vi "Main.vi"(11 "Module Admin":refnum<class "Delacor_lib_QMH_Module Admin.lvclass">) -> ()   [LabVIEW 2023, in "Graph_data_collector.lvlib"]
doc: "This template is based off of the Queued Message Handler design pattern and the Queued Message Handler project template that ships with LabVIEW.\n\nThe main difference is that the queue is private to this module and communication between modules is performed via Broadcast and Request events.\n\nRequest events are wrapped in public API methods and are handled in the Event Handling Loop (EHL) of this VI. Any module can register for Broadcast events sent by this module. The EHL generates messages based on user interface actions.\n\nThe Message Handling Loop (MHL) processes messages generated by the EHL, or by other messages. The messages are string values, so new messages can be added easily to the Message Cases case structure in the MHL. Each message cluster can also provide an optional value for Message Data, which is a variant that can be converted to whatever message-specific data is required.\n_____\nBased on DQMH Project Template 6.1.0.94."
uses:
  Graph_data_collector.lvlib
  <vilib>/Delacor/Delacor QMH/Libraries/Module Admin_class/Delacor_lib_QMH_Module Admin.lvclass
  Data Control.ctl
  Module Data--cluster.ctl
  <vilib>/Delacor/Delacor QMH/Libraries/Message Queue_class/Delacor_lib_QMH_Message Queue.lvclass/Delacor_lib_QMH_Message Queue.ctl
  Stop Argument--cluster.ctl
  <vilib>/Delacor/Delacor QMH/Libraries/Module Admin_class/Delacor_lib_QMH_Module Admin.lvclass/Delacor_lib_QMH_Module Admin.ctl
  New_Data Argument--cluster.ctl
  <vilib>/Utility/miscctls.llb/LVPointTypeDef.ctl
  Graph_UI/Module Data--cluster.ctl
  <vilib>/Delacor/Delacor QMH/Libraries/Message Queue_class/Delacor_lib_QMH_Enqueue Message (Single).vi
  <vilib>/Delacor/Delacor QMH/Libraries/Module Admin_class/Delacor_lib_QMH_Get External Launch.vi
  <vilib>/Utility/error.llb/Error Cluster From Error Code.vi
  <vilib>/ErrorRing/Error Ring.xnode
  <vilib>/Delacor/Delacor QMH/Libraries/Message Queue_class/Delacor_lib_QMH_Message Queue.lvclass
  Graph_UI/Graph_UI.lvlib
  Registration/Registration.lvlib
panel:
  in  "Data Type":T1 {"ЦАП, градС" format="%.3g"; "Тнагр, градС" format="%.3g"; "Q, мл" format="%.3g"; "Рдм, МПа" format="%.3g"; "Vпл, см3" format="Р2 %#.2f МПа"; "Рэфф, МПа" format="%.3g"; "dL, мм" format="%.4f"; "R, Ом" format="%.4f"; "Ргор, МПа" format="%.2f град.С"; "Рпл2, МПа" format="Р2 %#.2f МПа"; "Рпл1, МПа" format="Р2 %#.2f МПа"}
  in  "Clear_data":bool
  in  "Timeout":dbl=1.0 caption="Период" min=0.01 max=999.0 step=1.0 format="Период регистрации: %#.1f сек"
  in  "Select_OY":i32[](listbox)=[1] caption="Ось Y"
  in  "Select_OX":i32(listbox) caption="Ось Х"
  in  "Create_graph":bool
  out "error out":errorcluster
  out "Status":string
  in  "Simulate MHL Error":bool
  in  "Simulate EHL Error":bool
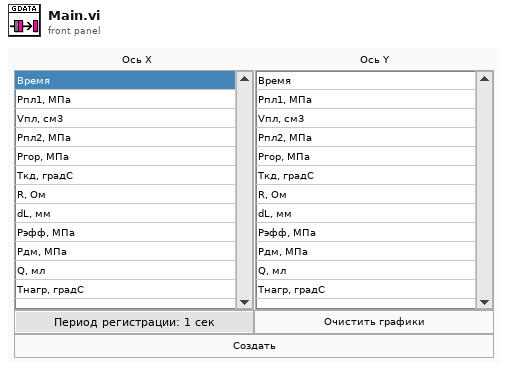
[diagram p1: front panel]
types:
  T1 = typedef "Graph_data_collector.lvlib/Data Control.ctl" = cluster{"Время":dbl, "Рпл1, МПа":dbl, "Vпл, см3":dbl, "Рпл2, МПа":dbl, "Ргор, МПа":dbl, "Ткд, градС":dbl, "R, Ом":dbl, "dL, мм":dbl, "Рэфф, МПа":dbl, "Рдм, МПа":dbl, "Q, мл":dbl, "Тнагр, градС":dbl, "ЦАП, градС":dbl}
  T2 = typedef "Graph_data_collector.lvlib/Request Events--cluster.ctl" = cluster{"Stop Module":refnum<user-event>, "Show Panel":refnum<user-event>, "Hide Panel":refnum<user-event>, "Get Module Execution Status":refnum<user-event>, "Show Diagram":refnum<user-event>, "New_Data":refnum<user-event>}
  T3 = typedef "Graph_data_collector.lvlib/Graph_UI.lvlib/Broadcast Events--cluster.ctl" = cluster{"Module Did Init":refnum<user-event>, "Status Updated":refnum<user-event>, "Error Reported":refnum<user-event>, "Module Did Stop":refnum<user-event>, "Update Module Execution Status":refnum<user-event>}
  T4 = typedef "Graph_data_collector.lvlib/Module Data--cluster.ctl" = cluster{"Status":string, "Array Lable":string[], "appended array":T1[], "Order Size":u32, "Graf_data_ref":refnum<vi>, "Actual_Data":T1}
  T5 = enum32{"invalid lock state", "Not Locked", "Locked (No Password)", "Password-protected"}
  T6 = typedef "Graph_data_collector.lvlib/Stop Argument--cluster.ctl" = cluster{"Origin":string, "Exit via Stop Module Req?":bool, "Wait for Module to stop?":bool}
  T7 = typedef "Graph_data_collector.lvlib/New_Data Argument--cluster.ctl" = cluster{"Graph_Data":T1}
  T8 = typedef "LVPointTypeDef.ctl" = cluster{"Horizontal":i16, "Vertical":i16}
  T9 = enum32{"Invalid", "Standard", "Closed", "Hidden", "Minimized", "Maximized"}
  T10 = typedef "Graph_data_collector.lvlib/Graph_UI.lvlib/Module Data--cluster.ctl" = cluster{"Status":string, "XY Graph our ref":refnum<vi>, "Array Lable":string[], "Ось Y":i32[], "Ось Х":i32, "Graph size":i32, "appended array":T1[], "XY Graph ref":refnum<vi>}
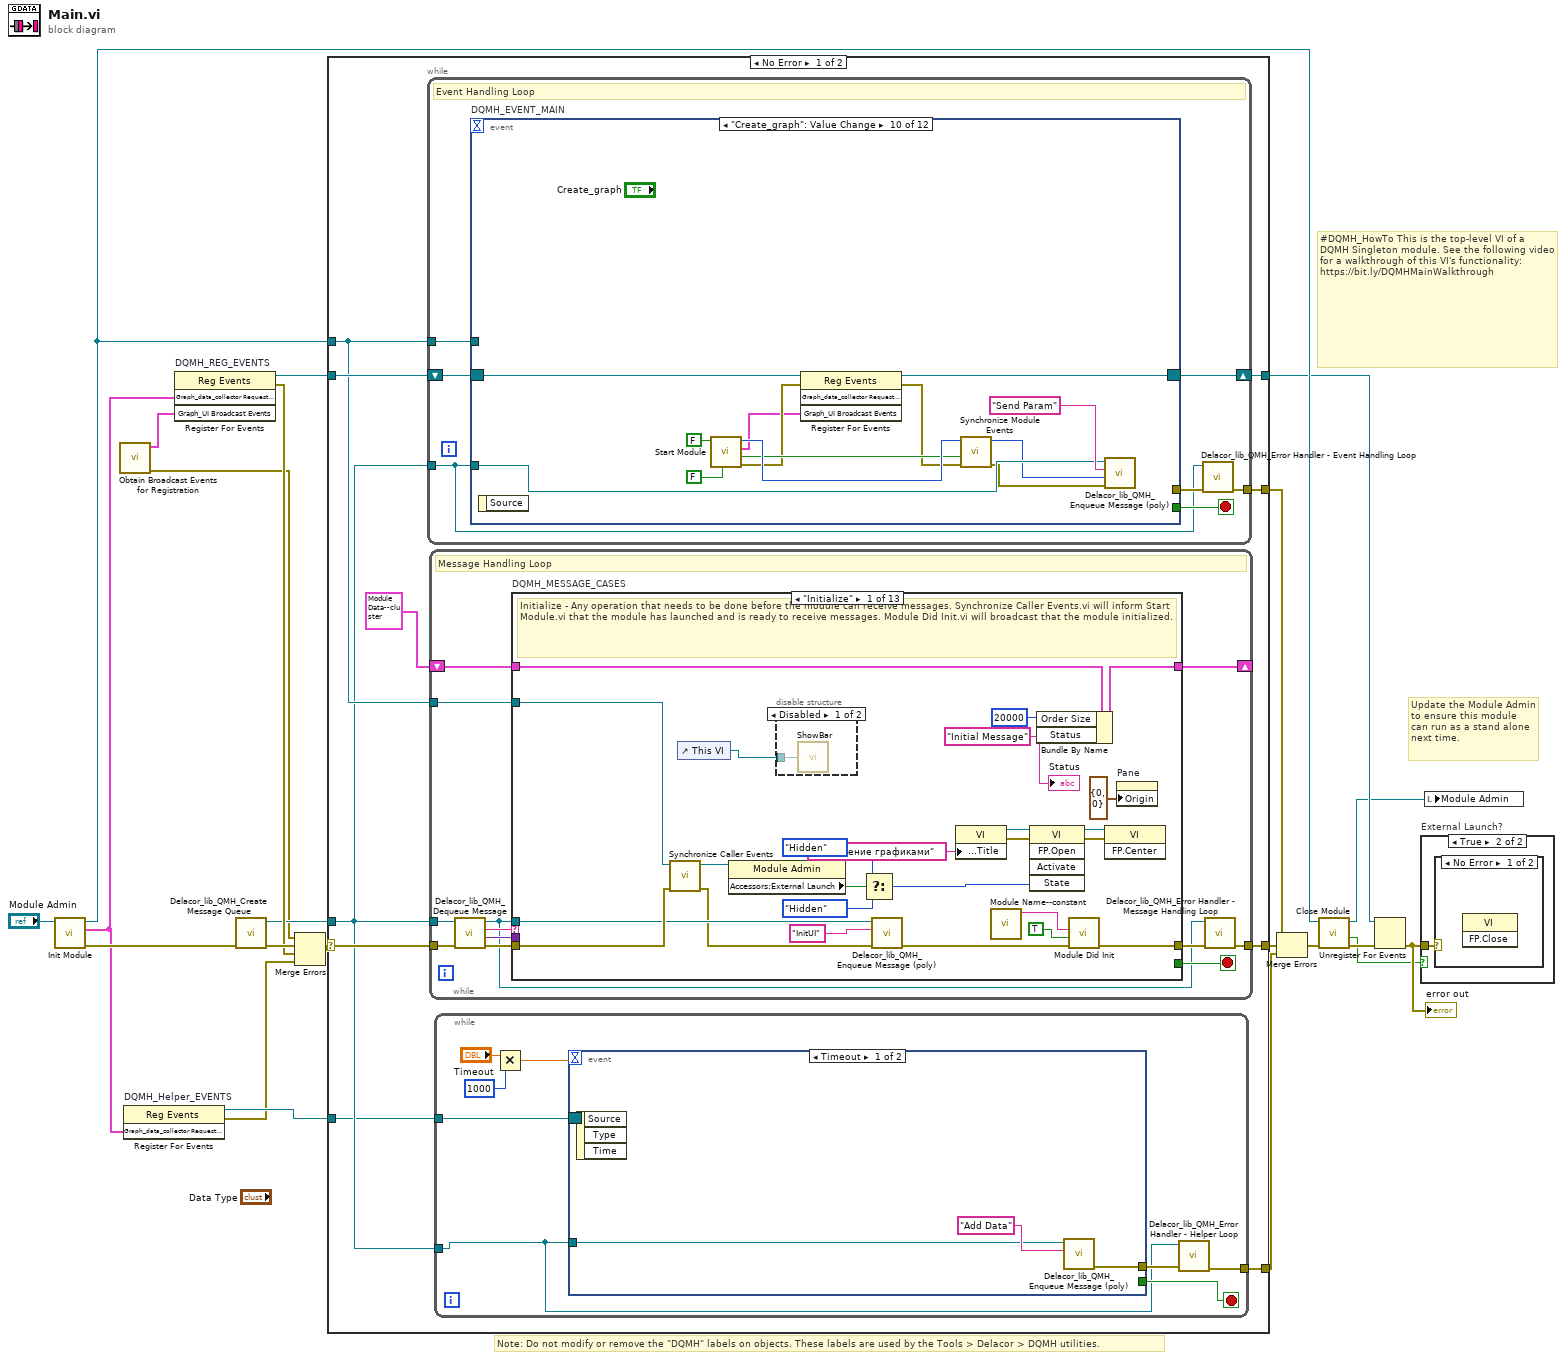
[diagram p0: block diagram]
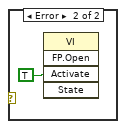
[diagram p3: hidden frame]
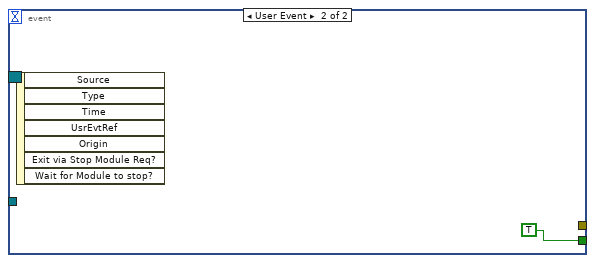
[diagram p4: hidden frame]
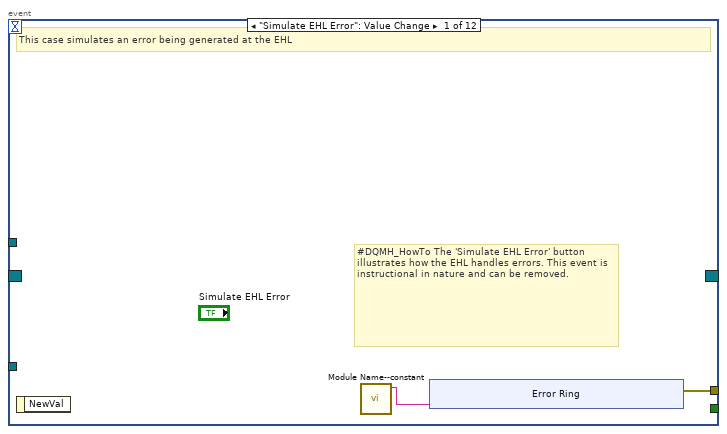
[diagram p5: hidden frame]
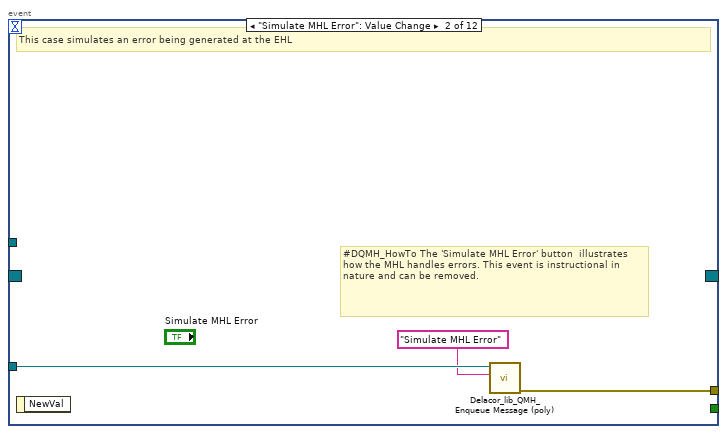
[diagram p6: hidden frame]
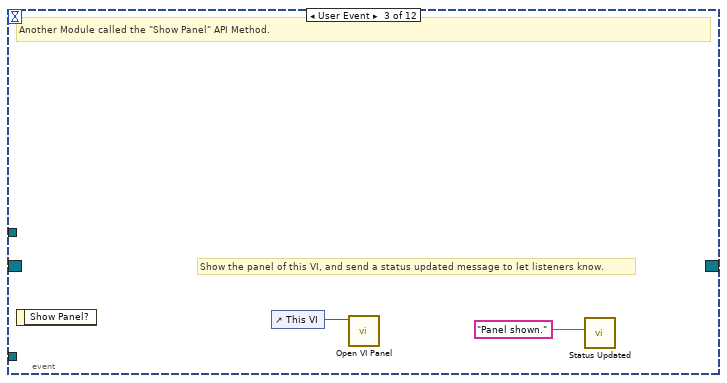
[diagram p7: hidden frame]
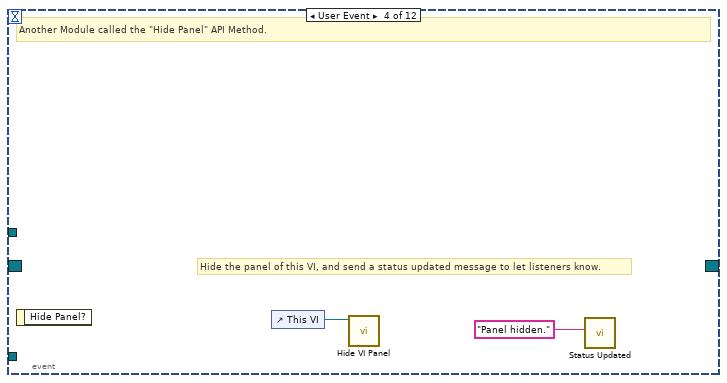
[diagram p8: hidden frame]
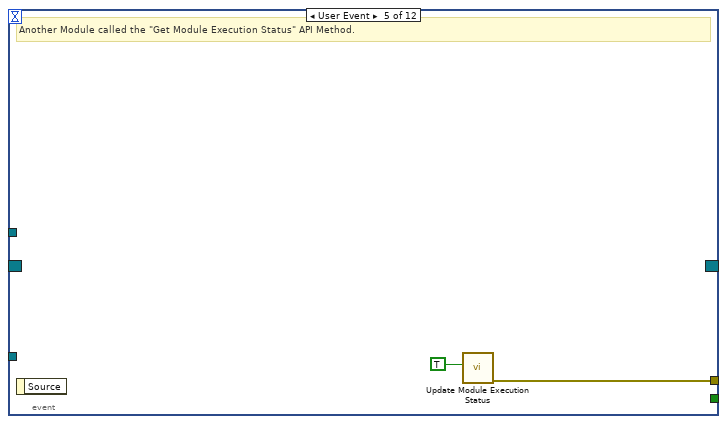
[diagram p9: hidden frame]
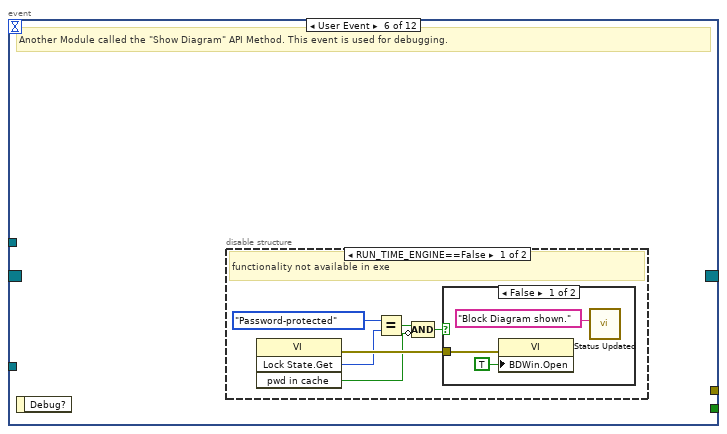
[diagram p10: hidden frame]
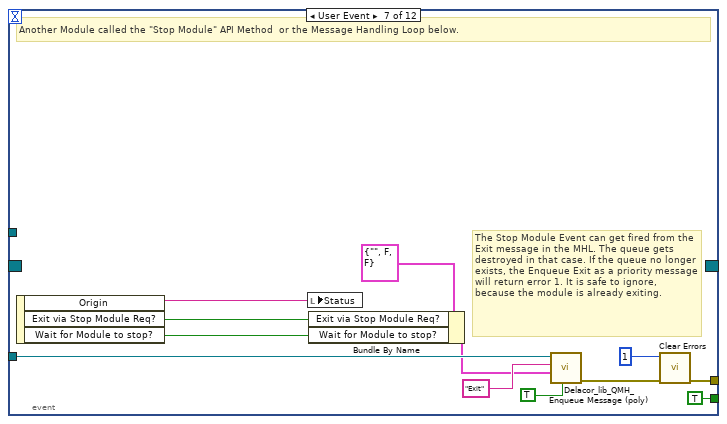
[diagram p13: hidden frame]
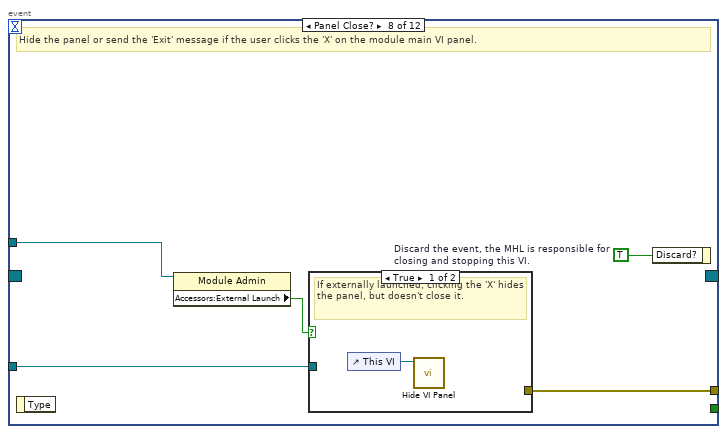
[diagram p14: hidden frame]
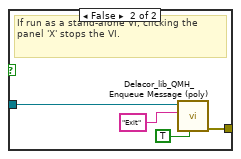
[diagram p15: hidden frame]
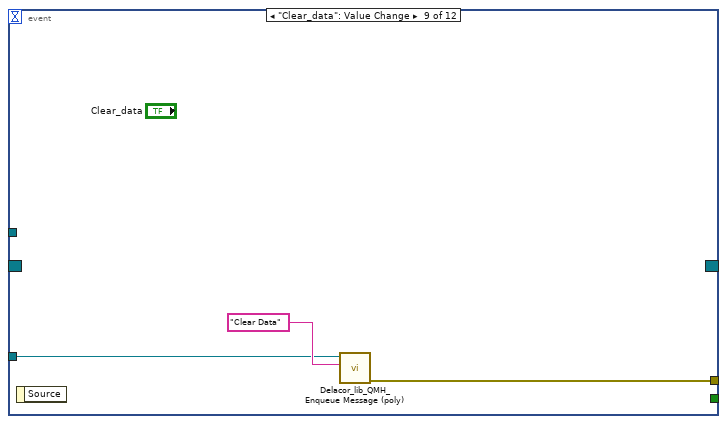
[diagram p16: hidden frame]
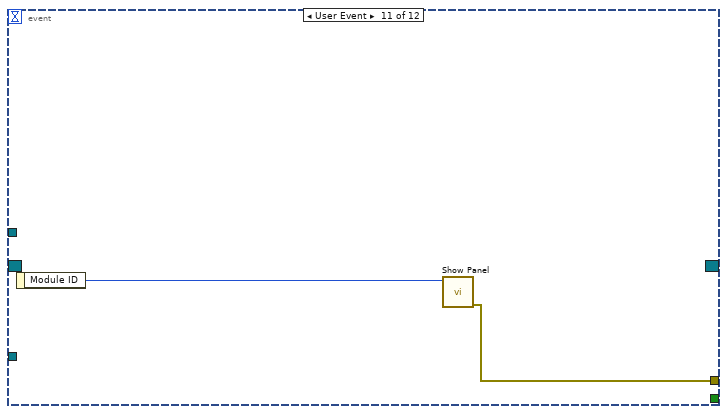
[diagram p17: hidden frame]
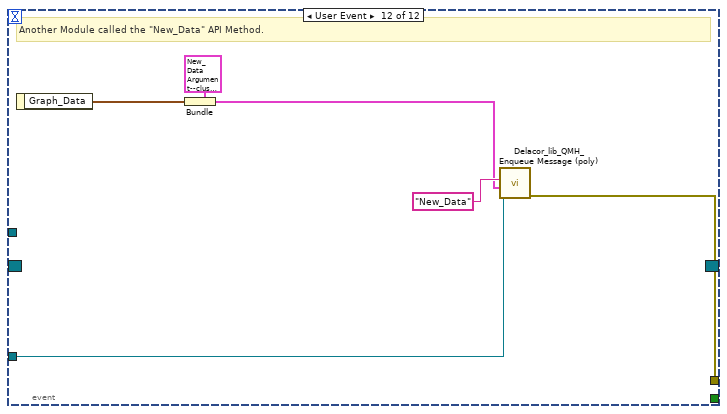
[diagram p18: hidden frame]
diagram:
  # "#DQMH_HowTo This is the top-level VI of a DQMH Singleton module. See the following video for a walkthrough of this VI's functionality: https://bit.ly/DQMHMainWalkthrough"
  # "Note: Do not modify or remove the \"DQMH\" labels on objects. These labels are used by the Tools > Delacor > DQMH utilities."
  # "Update the Module Admin to ensure this module can run as a stand alone next time."
  n1 = call "Init Module.vi"("Singleton Module Admin in"="Module Admin") -> ("error out"=w21:errorcluster, "Graph_data_collector Request Events"=w2:T2, "Singleton Module Admin out"=w13:refnum<class "Delacor_lib_QMH_Module Admin.lvclass">)  [unwired: 8 in]
  n2 = call "Obtain Broadcast Events for Registration.vi"() -> ("error out"=w5:errorcluster, "Graph_UI Broadcast Events"=w6:T3)  [unwired: 9 in, 1 out]
  n3 = register-events "DQMH_Helper_EVENTS"(w2) -> (reference out=w3:refnum<event-registration>, error out=w1:errorcluster)  [unwired: 2 in]
  n4 = register-events "DQMH_REG_EVENTS"(w2, w6) -> (reference out=w11:refnum<event-registration>, error out=w14:errorcluster)  [unwired: 2 in]
  n5 = call <vilib>:"Delacor_lib_QMH_Create Message Queue.vi"("error in"=w21) -> ("error out"=w16:errorcluster, "Message Queue"=w10:refnum<class "Delacor_lib_QMH_Message Queue.lvclass">)  [unwired: 9 in]
  n6 = Merge Errors(w5, w16, w14, w1) -> (w15:errorcluster)
  n7 = case shown="No Error" w15 {
    selector: w15 -> [w30 w288]
    tunnel: [w32 w287] -> w22
    tunnel: [w29 w293] -> w12
    tunnel: w11 -> [w28 w293]
    tunnel: w10 -> [w24 w286]
    tunnel: [w31 _] -> w19
    tunnel: w13 -> [w27 w289]
    tunnel: [w25 _] -> w4
    tunnel: w3 -> [w23 _]
    frame No Error {
      n8 = while {
        tunnel: w24 -> [w45]
        shift-right: [w48] -> w29
        shift-left: w28 -> [w49]
        tunnel: [w50] -> w31
        tunnel: w27 -> [w46]
        stop <- w47 stop-if-true
        # "Event Handling Loop"
        n9 = event "DQMH_EVENT_MAIN" shown="[9] \"Create_graph\": Value Change" {
          selector: w49 -> [_ _ _ _ _ _ _ _ _ w109 _ _]
          dyn-events: [_ _ _ _ _ _ _ _ _ w108 _ _] -> w48
          timeout: _ -> [_ _ _ _ _ _ _ _ _ _ _ _]
          tunnel: [_ _ _ _ _ _ TRUE ("Discard?") _ _ _ _ _] -> w47
          tunnel: w45 -> [_ w62 _ _ _ _ w86 w93 w101 w106 _ w124]
          tunnel: [w53 w63 _ _ w69 _ w89 w95 w102 _ w117 w119] -> w51
          tunnel: w46 -> [_ _ _ _ _ _ _ w92 _ _ _ _]
          event "Simulate EHL Error": Value Change {
            # "#DQMH_HowTo The 'Simulate EHL Error' button  illustrates how the EHL handles errors. This event is instructional in nature and can be removed."
            # "This case simulates an error being generated at the EHL"
            n10 = event-data() -> ()  [unwired: 1 in, 1 out]
            n11 = call "Module Name--constant.vi"() -> ("Module Name"=w52:string)  [unwired: 11 in]
            n12 = xnode "Error Ring"("parameter 0"=w52) -> ("error out"=w53:errorcluster)
          }
          event "Simulate MHL Error": Value Change {
            # "#DQMH_HowTo The 'Simulate MHL Error' button  illustrates how the MHL handles errors. This event is instructional in nature and can be removed."
            # "This case simulates an error being generated at the EHL"
            n13 = event-data() -> ()  [unwired: 1 in, 1 out]
            n14 = call-poly <vilib>:"Delacor_lib_QMH_Enqueue Message (poly).vi"("Message"="Simulate MHL Error", "Message Queue in"=w62) -> ("error out"=w63:errorcluster)  [unwired: 8 in, 1 out]
          }
          event User Event {
            # "Show the panel of this VI, and send a status updated message to let listeners know."
            # "Another Module called the \"Show Panel\" API Method."
            n15 = event-data() -> ()  [unwired: 1 in, 1 out]
            n16 = control-ref of="This VI"() -> (w65:refnum<vi>)
            n17 = call "Open VI Panel.vi"("VI"=w65) -> ()  [unwired: 10 in, 1 out]
            n18 = call "Status Updated.vi"("Status"="Panel shown." ("format string")) -> ()  [unwired: 10 in, 1 out]
          }
          event User Event {
            # "Hide the panel of this VI, and send a status updated message to let listeners know."
            # "Another Module called the \"Hide Panel\" API Method."
            n19 = event-data() -> ()  [unwired: 1 in, 1 out]
            n20 = control-ref of="This VI"() -> (w67:refnum<vi>)
            n21 = call "Hide VI Panel.vi"("VI"=w67) -> ()  [unwired: 10 in, 1 out]
            n22 = call "Status Updated.vi"("Status"="Panel hidden." ("format string")) -> ()  [unwired: 10 in, 1 out]
          }
          event User Event {
            # "Another Module called the \"Get Module Execution Status\" API Method."
            n23 = event-data() -> ()  [unwired: 1 in, 1 out]
            n24 = call "Update Module Execution Status.vi"("Running?"=TRUE) -> ("error out"=w69:errorcluster)  [unwired: 10 in]
          }
          event User Event {
            # "Another Module called the \"Show Diagram\" API Method. This event is used for debugging."
            n25 = event-data() -> ()  [unwired: 1 in, 1 out]
            n26 = disable-structure shown="RUN_TIME_ENGINE==False" {
              frame condition #0 (active) {
                # "functionality not available in exe"
                n27 = invoke class="VI" method="Lock State.Get"() -> (error out=w75:errorcluster, "Get Lock State"=w74:T5, "pwd in cache"=w71:bool)  [unwired: 4 in, 1 out]
                n28 = Equal?(x=T5."Password-protected", y=w74) -> (x = y?=w72:bool)
                n29 = Compound Arithmetic op=AND(w72, invert w71) -> (w70:bool)
                n30 = case shown="False" w70 {
                  tunnel: w75 -> [w78 _]
                  frame False {
                    n31 = property class="VI"(error in=w78, "BDWin.Open"=TRUE ("Block Diagram Window:Open")) -> ()  [unwired: 1 in, 2 out]
                    n32 = call "Status Updated.vi"("Status"="Block Diagram shown." ("format string")) -> ()  [unwired: 10 in, 1 out]
                  }
                  frame True {
                    # "Password-protected VI, and the password is not in the cache. Do not show the diagram."
                  }
                }
              }
              frame condition #1 {
              }
            }
          }
          event User Event {
            # "The Stop Module Event can get fired from the Exit message in the MHL. The queue gets destroyed in that case. If the queue no longer exists, the Enqueue Exit as a priority message will return error 1. It is safe to ignore, because the module is already exiting."
            # "Another Module called the \"Stop Module\" API Method  or the Message Handling Loop below."
            n33 = event-data() -> ("Origin"=w85:string, "Exit via Stop Module Req?"=w81:bool, "Wait for Module to stop?"=w80:bool)  [unwired: 1 in]
            n34 = local write "Status"(w85) -> ()
            n35 = Bundle By Name(cluster=T6 {"Origin"="", "Exit via Stop Module Req?"=FALSE, "Wait for Module to stop?"=FALSE} ("Stop Argument"), "Exit via Stop Module Req?"=w81, "Wait for Module to stop?"=w80) -> (w79:T6)
            n36 = call-poly <vilib>:"Delacor_lib_QMH_Enqueue Message (poly).vi"("Priority Message? (F)"=TRUE, "Message Data"=w79, "Message"="Exit", "Message Queue in"=w86) -> ("error out"=w90:errorcluster)  [unwired: 6 in, 1 out]
            n37 = call <vilib>:"Clear Errors.vi"("error in (no error)"=w90, "specific error code to clear (0: all)"=1) -> ("error out"=w89:errorcluster)  [unwired: 4 in, 1 out]
          }
          event Panel Close? {
            w94 = TRUE  # Discard the event, the MHL is responsible for closing and stopping this VI.
            # "Hide the panel or send the 'Exit' message if the user clicks the 'X' on the module main VI panel."
            n38 = event-data() -> ()  [unwired: 1 in, 1 out]
            n39 = property class="Module Admin"(reference=w92) -> ("Accessors:External Launch"=w91:bool)  [unwired: 1 in, 2 out]
            n40 = case shown="True" w91 {
              tunnel: w93 -> [_ w99]
              tunnel: [_ w100] -> w95
              frame True {
                # "If externally launched, clicking the 'X' hides the panel, but doesn't close it."
                n41 = control-ref of="This VI"() -> (w96:refnum<vi>)
                n42 = call "Hide VI Panel.vi"("VI"=w96) -> ()  [unwired: 10 in, 1 out]
              }
              frame False {
                # "If run as a stand-alone VI, clicking the panel 'X' stops the VI."
                n43 = call-poly <vilib>:"Delacor_lib_QMH_Enqueue Message (poly).vi"("Priority Message? (F)"=TRUE, "Message"="Exit", "Message Queue in"=w99) -> ("error out"=w100:errorcluster)  [unwired: 7 in, 1 out]
              }
            }
            n44 = event-data("Discard?"=w94) -> ()  [unwired: 1 in, 1 out]
          }
          event "Clear_data": Value Change {
            n45 = event-data() -> ()  [unwired: 1 in, 1 out]
            n46 = call-poly <vilib>:"Delacor_lib_QMH_Enqueue Message (poly).vi"("Message"="Clear Data", "Message Queue in"=w101) -> ("error out"=w102:errorcluster)  [unwired: 8 in, 1 out]
          }
          event "Create_graph": Value Change {
            n47 = event-data() -> ()  [unwired: 1 in, 1 out]
            n48 = call "Start Module.vi"("Show Main VI Diagram on Init (F)"=FALSE, "Run as Singleton? (F)"=FALSE) -> ("error out"=w114:errorcluster, "Wait for Event Sync?"=w115:bool, "Graph_UI Broadcast Events"=w110:T3, "Module ID"=w116:i32)  [unwired: 6 in]
            n49 = register-events(reference=w109, error in=w114, w110) -> (reference out=w108:refnum<event-registration>, error out=w113:errorcluster)  [unwired: 1 in]
            n50 = call "Synchronize Module Events.vi"("error in"=w113, "Wait for Event Sync?"=w115, "Module ID in"=w116) -> ("error out"=w105:errorcluster, "Module ID out"=w104:i32)  [unwired: 7 in]
            n51 = call-poly <vilib>:"Delacor_lib_QMH_Enqueue Message (poly).vi"("error in"=w105, "Message Data"=w104, "Message"="Send Param", "Message Queue in"=w106) -> ()  [unwired: 6 in, 2 out]
          }
          event User Event {
            n52 = event-data() -> ("Module ID"=w118:i32)  [unwired: 1 in]
            n53 = call "Show Panel.vi"("Module ID"=w118) -> ("error out"=w117:errorcluster)  [unwired: 10 in]
          }
          event User Event {
            # "Another Module called the \"New_Data\" API Method."
            n54 = event-data() -> ("Graph_Data"=w120:T1)  [unwired: 1 in]
            n55 = Bundle(cluster=T7 {"Graph_Data"={"Время"=0.0, "Рпл1, МПа"=0.0, "Vпл, см3"=0.0, "Рпл2, МПа"=0.0, "Ргор, МПа"=0.0, "Ткд, градС"=0.0, "R, Ом"=0.0, "dL, мм"=0.0, "Рэфф, МПа"=0.0, "Рдм, МПа"=0.0, "Q, мл"=0.0, "Тнагр, градС"=0.0, "ЦАП, градС"=0.0}} ("New_Data Argument"), "Graph_Data"=w120) -> (w121:T7)
            n56 = call-poly <vilib>:"Delacor_lib_QMH_Enqueue Message (poly).vi"("Message Data"=w121, "Message"="New_Data", "Message Queue in"=w124) -> ("error out"=w119:errorcluster)  [unwired: 7 in, 1 out]
          }
        }
        n57 = call-dynamic "Delacor_lib_QMH_Error Handler - Event Handling Loop.vi"("error in"=w51, "Message Queue in"=w45) -> ("dup error in"=w50:errorcluster)  [unwired: 8 in, 1 out]
      }
      n58 = while {
        tunnel: w24 -> [w127]
        shift-right: [w131] -> _
        shift-left: T4 {"Status"="", "Array Lable"=[], "appended array"=[], "Order Size"=0, "Graf_data_ref"=refnum, "Actual_Data"={"Время"=0.0, "Рпл1, МПа"=0.0, "Vпл, см3"=0.0, "Рпл2, МПа"=0.0, "Ргор, МПа"=0.0, "Ткд, градС"=0.0, "R, Ом"=0.0, "dL, мм"=0.0, "Рэфф, МПа"=0.0, "Рдм, МПа"=0.0, "Q, мл"=0.0, "Тнагр, градС"=0.0, "ЦАП, градС"=0.0}} ("Data Cluster") -> [w132]
        tunnel: w30 -> [w135]
        tunnel: [w133] -> w32
        tunnel: w27 -> [w125]
        stop <- w130 stop-if-true
        # "Message Handling Loop"
        n59 = call-dynamic "Delacor_lib_QMH_Dequeue Message.vi"("error in"=w135, "Message Queue in"=w127) -> ("error out"=w134:errorcluster, "Message Data"=w128:variant, "Message"=w129:string, "Message Queue out"=w126:refnum<class "Delacor_lib_QMH_Message Queue.lvclass">)  [unwired: 6 in]
        n60 = case "DQMH_MESSAGE_CASES" shown="\"Initialize\"" w129 {
          selector: w129 -> [_ _ _ _ _ _ _ _ _ _ _ _ w273]
          tunnel: w126 -> [w143 _ _ _ _ _ _ _ _ _ w240 w265 _]
          tunnel: w134 -> [w159 w164 w172 w175 w183 w195 w197 w220 w225 w230 w247 w271 w275]
          tunnel: [w158 w164 w170 w174 w190 w194 w210 w219 w225 w229 w243 w268 w276] -> w136
          tunnel: w132 -> [w150 w163 w171 w173 w180 w193 w208 w217 w224 w227 w242 w264 w274]
          tunnel: [w149 w163 w166 w173 w180 w192 w202 w218 w224 w227 w242 w264 w274] -> w131
          tunnel: [_ _ _ _ _ _ _ _ _ _ _ w263 _] -> w130
          tunnel: w128 -> [_ _ w169 _ w182 _ _ _ _ _ w241 w262 _]
          tunnel: w125 -> [w151 _ _ _ _ _ _ _ _ _ w239 w257 _]
          frame "Initialize" {
            w145 = "Initial Message" ("Initial Message")
            # "Initialize - Any operation that needs to be done before the module can receive messages. Synchronize Caller Events.vi will inform Start Module.vi that the module has launched and is ready to receive messages. Module Did Init.vi will broadcast that the module initialized."
            n61 = call "Synchronize Caller Events.vi"("error in (no error)"=w159, "Singleton Module Admin in"=w151) -> ("error out"=w142:errorcluster, "Singleton Module Admin out"=w146:refnum<class "Delacor_lib_QMH_Module Admin.lvclass">)  [unwired: 8 in]
            n62 = control-ref of="This VI"() -> (w138:refnum<vi>)
            n63 = property class="Module Admin"(reference=w146) -> ("Accessors:External Launch"=w155:bool)  [unwired: 1 in, 2 out]
            n64 = disable-structure shown="Disabled" {
              disable-tunnel: w138 -> [w162 _]
              frame Disabled {
                n65 = call "ShowBar.vi"("This VI"=w162) -> ()
              }
              frame Enabled {
              }
            }
            n66 = Select(t=T9."Hidden" ("State"), s=w155, f=T9."Hidden" ("State")) -> (s? t:f=w152:T9)
            n67 = call-poly <vilib>:"Delacor_lib_QMH_Enqueue Message (poly).vi"("error in"=w142, "Message"="InitUI", "Message Queue in"=w143) -> ("error out"=w141:errorcluster)  [unwired: 7 in, 1 out]
            n68 = property class="VI"("Front Panel.Title"="Управление графиками" ("Front Panel Window:Title")) -> (reference out=w157:refnum<vi>, error out=w161:errorcluster)  [unwired: 2 in]
            n69 = call "Module Name--constant.vi"() -> ("Module Name"=w147:string)  [unwired: 11 in]
            n70 = invoke class="VI" method="FP.Open"(reference=w157, error in=w161, "State"=w152) -> (reference out=w156:refnum<vi>, error out=w160:errorcluster)  [unwired: 2 in, 3 out]
            n71 = Bundle By Name(cluster=w150, "Order Size"=u32 20000, "Status"=w145) -> (w149:T4)
            n72 = call "Module Did Init.vi"("error in (no error)"=w141, "Initialized?"=TRUE, "Origin"=w147) -> ("error out"=w158:errorcluster)  [unwired: 8 in]
            n73 = invoke class="VI" method="FP.Center"(reference=w156, error in=w160) -> ()  [unwired: 1 in, 3 out]
            n74 = property on="Pane" class="Pane"("Origin"=T8 {"Horizontal"=0, "Vertical"=0}) -> ()  [unwired: 2 in, 2 out]
            "Status" <- w145
          }
          frame "---Module Specific---" {
            # "Separator -- The following cases handle messages specific to this Module."
          }
          frame "New_Data" {
            n75 = Variant To Data(error in=w172, type=T7 {"Graph_Data"={"Время"=0.0, "Рпл1, МПа"=0.0, "Vпл, см3"=0.0, "Рпл2, МПа"=0.0, "Ргор, МПа"=0.0, "Ткд, градС"=0.0, "R, Ом"=0.0, "dL, мм"=0.0, "Рэфф, МПа"=0.0, "Рдм, МПа"=0.0, "Q, мл"=0.0, "Тнагр, градС"=0.0, "ЦАП, градС"=0.0}} ("New_Data Argument"), Variant=w169) -> (data=w167:T7, error out=w170:errorcluster)
            n76 = Unbundle By Name(w167) -> ("Graph_Data"=w165:T1)
            n77 = Bundle By Name(cluster=w171, "Actual_Data"=w165) -> (w166:T4)
          }
          frame "---Copy This Frame---" {
            # "Duplicate this frame when creating new messages.  Change this comment in the duplicated frame to describe this message."
            n78 = Merge Errors(w175) -> (w174:errorcluster)
          }
          frame "Send Param" {
            # "Duplicate this frame when creating new messages.  Change this comment in the duplicated frame to describe this message."
            n79 = Unbundle By Name(w180) -> ("appended array"=w187:T1[], "Order Size"=w188:u32, "Array Lable"=w189:string[])
            n80 = Variant To Data(error in=w183, type=0 ("Module ID out"), Variant=w182) -> (data=w177:i32, error out=w178:errorcluster)
            n81 = Bundle By Name(cluster=T10 {"Status"="", "XY Graph our ref"=refnum, "Array Lable"=[], "Ось Y"=[], "Ось Х"=0, "Graph size"=20000, "appended array"=[], "XY Graph ref"=refnum} ("Module Data"), "Ось Х"="Select_OX", "Ось Y"="Select_OY", "appended array"=w187, "Graph size"=w188, "Array Lable"=w189) -> (w179:T10)
            n82 = call "SetP.vi"("error in"=w178, "Module Data"=w179, "Module ID"=w177) -> ("error out"=w176:errorcluster)  [unwired: 8 in]
            n83 = Merge Errors(w176) -> (w190:errorcluster)
          }
          frame "Clear Data" {
            # "Duplicate this frame when creating new messages.  Change this comment in the duplicated frame to describe this message."
            n84 = Bundle By Name(cluster=w193, "appended array"=T1[] []) -> (w192:T4)
            n85 = Merge Errors(w195) -> (w194:errorcluster)
          }
          frame "Add Data" {
            # "Duplicate this frame when creating new messages.  Change this comment in the duplicated frame to describe this message."
            n86 = Get Date/Time In Seconds() -> (seconds since 1Jan1904=w207:timestamp)
            n87 = Unbundle By Name(w208) -> ("appended array"=w203:T1[], "Order Size"=w204:u32, "Actual_Data"=w196:T1)
            n88 = To Double Precision Float(number=w207) -> (double precision float=w206:dbl)
            n89 = Bundle By Name(cluster=w196, "Время"=w206) -> (w205:T1)
            n90 = call "Order_Size_Control.vi"("New Data"=w205, "Order Size"=w204, "Old Array"=w203) -> ("New Data"=w200:T1, "New Array"=w201:T1[])  [unwired: 7 in]
            n91 = Bundle By Name(cluster=w208, "appended array"=w201) -> (w202:T4)
            n92 = call "New Data.vi"("error in"=w197, "Data"=w200, "Module ID"=-1) -> ("error out"=w199:errorcluster)  [unwired: 8 in]
            n93 = call <vilib>:"Clear Errors.vi"("error in (no error)"=w199) -> ("error out"=w198:errorcluster)  [unwired: 5 in, 1 out]
            n94 = Merge Errors(w198) -> (w210:errorcluster)
          }
          frame "InitUI" {
            # "Duplicate this frame when creating new messages.  Change this comment in the duplicated frame to describe this message."
            n95 = control-ref of="Data Type"() -> (w211:refnum<vi>)
            n96 = call "Init_UI.vi"("Data ref"=w211) -> ("error out"=w216:errorcluster, "Array Labels"=w215:string[])  [unwired: 9 in]
            n97 = Bundle By Name(cluster=w217, "Array Lable"=w215) -> (w218:T4)
            n98 = property on="Select_OX" class="LstBox (strict)"(error in=w216, "Item Names"=w215) -> (error out=w214:errorcluster)  [unwired: 1 in, 1 out]
            n99 = property on="Select_OY" class="LstBox (strict)"(error in=w214, "Item Names"=w215) -> (error out=w213:errorcluster)  [unwired: 1 in, 1 out]
            n100 = disable-structure shown="Enabled" {
              disable-tunnel: w213 -> [w222 w223]
              disable-tunnel: [w221 w223] -> w212
              frame Disabled {
                n101 = call "Show Panel.vi"("error in (no error)"=w222) -> ("error out"=w221:errorcluster)  [unwired: 10 in]
              }
              frame Enabled {
              }
            }
            n102 = Merge Errors(w212, w220) -> (w219:errorcluster)
          }
          frame "---Exit and Error Handling---" {
            # "Separator - The following cases handle errors and exit messages."
          }
          frame "Simulate MHL Error" {
            # "#DQMH_HowTo The 'Simulate MHL Error' button  illustrates how the MHL handles errors. This event is instructional in nature and can be removed."
            # "Simulate an error occurring at the MHL"
            n103 = call "Module Name--constant.vi"() -> ("Module Name"=w226:string)  [unwired: 11 in]
            n104 = xnode "Error Ring"("parameter 0"=w226) -> ("error out"=w228:errorcluster)
            n105 = Merge Errors(w230, w228) -> (w229:errorcluster)
          }
          frame "Error" {
            # "#CodeRecommended - If you ever change the name of this \"Error\" message, you'll need to update the name in the Check Loop Error.vi as well."
            # "#CodeRecommended - If the module is running in standalone mode (External Launch = FALSE), this code will pop up an error dialog and call the 'Exit' message if an error occurs. Add more fine-grained error handling here."
            # "Error - Check the error message data and respond accordingly. This message is sent by the \"Error Handler\" VIs at the end of each loop in this application."
            n106 = property class="Module Admin"(reference=w239) -> ("Accessors:External Launch"=w238:bool)  [unwired: 1 in, 2 out]
            n107 = Variant To Data(error in=w247, type=errorcluster {"status"=FALSE, "code"=0, "source"=""} ("error constant"), Variant=w241) -> (data=w248:errorcluster, error out=w245:errorcluster)
            n108 = call "Error Reported.vi"("Error"=w248) -> ()  [unwired: 10 in, 1 out]
            n109 = case shown="True" w238 {
              tunnel: [w253 _] -> w244
              tunnel: w240 -> [w251 _]
              tunnel: w248 -> [w252 _]
              frame False {
                # "If the module is running standalone, then pop up an error dialog and call the \"Exit\" message."
                n110 = call <vilib>:"Simple Error Handler.vi"("error in (no error)"=w252) -> ()  [unwired: 4 in, 5 out]
                n111 = call-poly <vilib>:"Delacor_lib_QMH_Enqueue Message (poly).vi"("Priority Message? (F)"=TRUE, "Message"="Exit", "Message Queue in"=w251) -> ("error out"=w253:errorcluster)  [unwired: 7 in, 1 out]
              }
              frame True {
                # "If the module was launched externally, calling the Error Reported broadcast VI is the only action performed by the \"Error\" message. The module's caller can then process the error appropriately."
              }
            }
            n112 = Merge Errors(w245, w244) -> (w243:errorcluster)
            n113 = local write "error out"(w243) -> ()
          }
          frame "Exit" {
            w261 = 91  # 91: not all Exit messages will have an argument
            w263 = TRUE  # Stop the VI
            # "Release the message queue reference"
            # "Exit - Exit the application."
            n114 = Variant To Data(error in=w271, type=T6 {"Origin"="", "Exit via Stop Module Req?"=FALSE, "Wait for Module to stop?"=FALSE} ("Stop Argument"), Variant=w262) -> (data=w259:T6, error out=w267:errorcluster)
            n115 = call <vilib>:"Clear Errors.vi"("error in (no error)"=w267, "specific error code to clear (0: all)"=w261) -> ("error out"=w270:errorcluster)  [unwired: 4 in, 1 out]
            n116 = control-ref of="This VI"() -> (w258:refnum<vi>)
            n117 = call-dynamic "Delacor_lib_QMH_Release Message Queue.vi"("error in"=w270, "Message Queue"=w265) -> ("error out"=w269:errorcluster)  [unwired: 9 in]
            n118 = call "Handle Exit.vi"("Stop Argument"=w259, "Admin in"=w257, "VI reference"=w258) -> ("error out"=w266:errorcluster)  [unwired: 7 in, 1 out]
            n119 = call "Stop Module.vi"("Origin"="Graph_UI Tester sent Stop Message", "Module ID"=-1) -> ("error out"=w254:errorcluster)  [unwired: 9 in]
            n120 = Merge Errors(w254, w269, w266) -> (w268:errorcluster)
          }
          frame Default {
            # "'Default' case only runs if there is a message that isn't defined in any of the other cases.  Output a programming error."
            n121 = call "Module Name--constant.vi"() -> ("Module Name"=w272:string)  [unwired: 11 in]
            n122 = xnode "Error Ring"("parameter 0"=w273, "parameter 1"=w272) -> ("error out"=w277:errorcluster)
            n123 = Merge Errors(w275, w277) -> (w276:errorcluster)
          }
        }
        n124 = call-dynamic "Delacor_lib_QMH_Error Handler - Message Handling Loop.vi"("error in"=w136, "Message Queue in"=w126) -> ("dup error in"=w133:errorcluster)  [unwired: 8 in, 1 out]
      }
      n125 = while {
        tunnel: [w40] -> w25
        tunnel: w24 -> [w33]
        tunnel: w23 -> [w35]
        stop <- w34 stop-if-true
        n126 = Multiply(x="Timeout", y=u32 1000) -> (x*y=w37:dbl)
        n127 = event shown="[0] Timeout" {
          selector: w35 -> [_ _]
          dyn-events: _ -> [_ _]
          timeout: w37 -> [_ _]
          tunnel: [w42 _] -> w36
          tunnel: w33 -> [w41 _]
          tunnel: [_ TRUE] -> w34
          event Timeout {
            n128 = event-data() -> ()  [unwired: 1 in, 3 out]
            n129 = call-poly <vilib>:"Delacor_lib_QMH_Enqueue Message (poly).vi"("Message"="Add Data", "Message Queue in"=w41) -> ("error out"=w42:errorcluster)  [unwired: 8 in, 1 out]
          }
          event User Event {
            n130 = event-data() -> ()  [unwired: 1 in, 7 out]
          }
        }
        n131 = call-dynamic "Delacor_lib_QMH_Error Handler - Helper Loop.vi"("error in"=w36, "Message Queue in"=w33) -> ("dup error in"=w40:errorcluster)  [unwired: 8 in, 1 out]
      }
    }
    frame Error {
      # "Synchronize Caller Events.vi will inform Start Module.vi that the module has launched and will let the code calling Start Module.vi register for broadcasts and would permit the caller receive the broadcast that an error occurred at launch time."
      n132 = call-dynamic "Delacor_lib_QMH_Release Message Queue.vi"("error in"=w288, "Message Queue"=w286) -> ("error out"=w287:errorcluster)  [unwired: 9 in]
      n133 = call "Synchronize Caller Events.vi"("Singleton Module Admin in"=w289) -> ("error out"=w294:errorcluster)  [unwired: 9 in, 1 out]
      n134 = call "Module Name--constant.vi"() -> ("Module Name"=w292:string)  [unwired: 11 in]
      n135 = Format Into String(format string="An error occurred during initialization. %s is no longer running.", w292) -> (resulting string=w290:string)  [unwired: 2 in, 1 out]
      n136 = Merge Errors(w287, w294) -> (w295:errorcluster)
      n137 = call "Error Reported.vi"("Additional Information"=w290, "Error"=w295) -> ()  [unwired: 9 in, 1 out]
    }
  }
  n138 = Merge Errors(w19, w22, w4) -> (w18:errorcluster)
  n139 = call "Close Module.vi"("error in (no error)"=w18, "Module Admin in"=w13) -> ("error out"=w20:errorcluster, "External Launch"=w7:bool, "Module Admin out"=w8:refnum<class "Delacor_lib_QMH_Module Admin.lvclass">)  [unwired: 7 in]
  n140 = Unregister For Events(event registration refnum=w12, error in=w20) -> (error out=w17:errorcluster)
  "error out" <- w17
  n141 = case "External Launch?" shown="True" w7 {
    tunnel: w17 -> [_ w296]
    frame False {
    }
    frame True {
      n142 = case shown="No Error" w296 {
        frame No Error {
          n143 = invoke class="VI" method="FP.Close"() -> ()  [unwired: 3 in, 3 out]
        }
        frame Error {
          n144 = invoke class="VI" method="FP.Open"("Activate"=TRUE ("Activate?")) -> ()  [unwired: 4 in, 5 out]
        }
      }
    }
  }
  n145 = local write "Module Admin"(w8) -> ()
